vi "locate U8.vi"(8 "error in":errorcluster, 10 "name":string, 11 "data dictionary in":refnum<class "data dictionary.lvclass">) -> (0 "error out":errorcluster, 2 "index":i32, 3 "data dictionary out":refnum<class "data dictionary.lvclass">)   [LabVIEW 2013, in "tag bus.lvlib" / "data dictionary.lvclass"]
doc: "Locates a tag within the dictionary and provides its index within the associated data table."
uses:
  data dictionary.lvclass
  tag/Data Type.ctl
  tag/tag descriptor.lvclass
  tag bus.lvlib
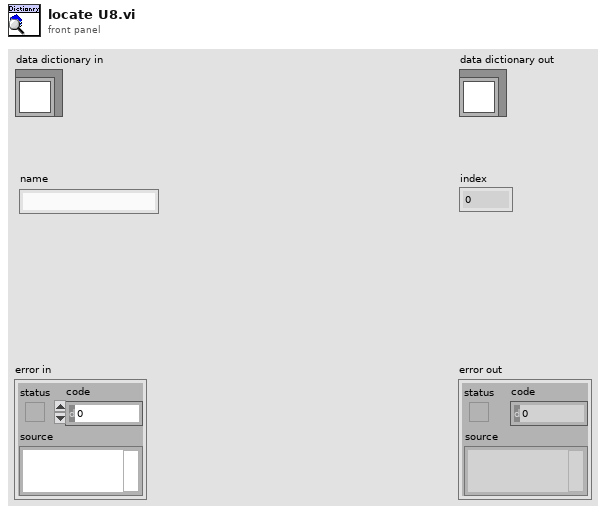
[diagram p1: front panel]
types:
  T1 = typedef "tag bus.lvlib/tag descriptor.lvclass/Data Type.ctl" = enum16{"Double", "Single", "I64", "I32", "I16", "I8", "U64", "U32", "U16", "U8", "Boolean", "String", "Array of Double", "Array of Single", "Array of I64", "Array of I32", "Array of I16", "Array of I8", "Array of U64", "Array of U32", "Array of U16", "Array of U8", "Array of Boolean", "Array of String"}
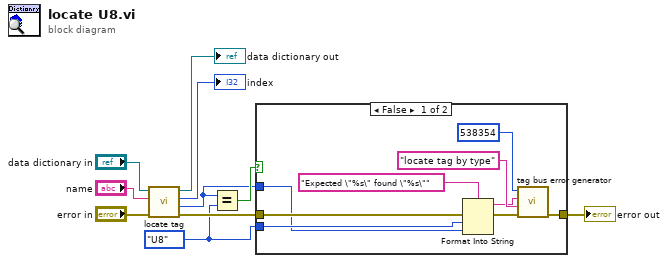
[diagram p0: block diagram]
diagram:
  w2 = Data_Type."U8" ("y")
  n1 = call "locate tag.vi"("error in"="error in", "name"="name", "data dictionary in"="data dictionary in") -> ("error out"=w3:errorcluster, "data type"=w1:T1, "index"=→"index":i32, "data dictionary out"=→"data dictionary out":refnum<class "data dictionary.lvclass">)  [unwired: 5 in]
  n2 = Equal?(x=w1, y=w2) -> (x = y?=w5:bool)
  n3 = case shown="False" w5 {
    tunnel: [w18 w20] -> w4
    tunnel: w3 -> [w19 w20]
    tunnel: w2 -> [w13 _]
    tunnel: w1 -> [w12 _]
    frame False {
      n4 = Format Into String(format string="Expected \"%s\" found \"%s\"", error in=w19, w13, w12) -> (resulting string=w14:string, error out=w15:errorcluster)  [unwired: 1 in]
      n5 = call "tag bus error generator.vi"("error in"=w15, "source"="locate tag by type", "append error message"=w14, "error code (0)"=538354) -> ("error out"=w18:errorcluster)  [unwired: 5 in]
    }
    frame True {
    }
  }
  "error out" <- w4
